vi "Create_Destination_for_Duplicate.vi"(8 "error in (no error)":errorcluster, 9 "subDirectory":string="data", 10 "Destinations in":refnum<class "AB_Destination.lvclass">[](array[class]), 11 "AB_Source_Library in":refnum<class "AB_Source_Library.lvclass">) -> (0 "error out":errorcluster, 1 "newPath":path, 2 "Destinations out":refnum<class "AB_Destination.lvclass">[](array[class]), 3 "AB_Source_Library out":refnum<class "AB_Source_Library.lvclass">)   [LabVIEW 2020, in "AB_Source_Library.lvclass"]
uses:
  <vilib>/AppBuilder/AB_Classes/Source/Library/AB_Source_Library.lvclass
  <vilib>/AppBuilder/AB_Classes/Destination/AB_Destination.lvclass
  e:/builds/penguin/labview/branches/2020/dev/dist/vi.lib/AppBuilder/AB_Classes/Source/AB_Source.lvclass
  <vilib>/AppBuilder/AB_Classes/Source/AB_Source.lvclass
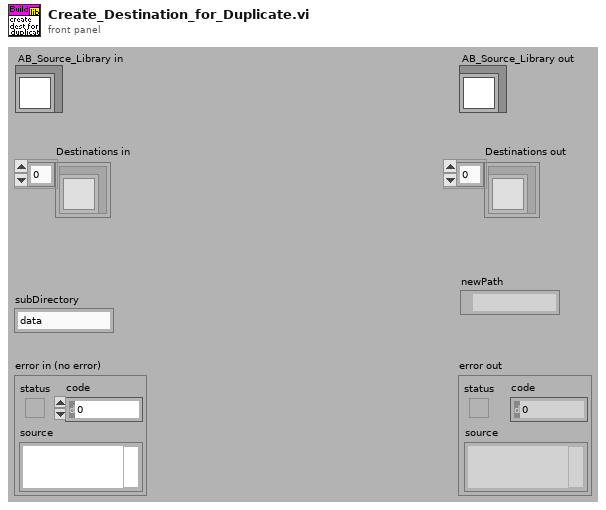
[diagram p1: front panel]
types:
  T1 = typedef "AB_Source.ctl" = cluster{"path":path, "itemID":string, "parentIndex":i32, "sourceInclusion":T2, "destinationIndex":i32, "properties":T3[], "newName":string, "lvfile":bool, "valid":bool, "eng_inBuild":bool, "eng_isNonVILink":bool, "Amalgamation":bool, "Amalgamation Piece":bool, "eng_delimitedName":string, "preventRename":bool}
  T2 = typedef "AB_Source_Inclusion.ctl" = enum16{"IncludeIfReferenced", "Include", "Exclude", "TopLevel"}
  T3 = typedef "AB_Source_Properties.ctl" = cluster{"sourcePropertyType":T4, "value":variant}
  T4 = typedef "AB_Source_Property_Type.ctl" = enum16{"Remove block diagram", "Remove front panel", "Password", "Window has title bar", "Show menu bar", "Show vertical scroll bar", "Show horizontal scroll bar", "Show toolbar", "Show Abort button", "Show fp when called", "Window behavior", "Allow user to close window", "Window run-time position", "Run when opened", "Allow debugging", "Auto error handling", "Generate guard code", "Use stack variables", "Expression folding", "Integer only", "Inline subVI"}
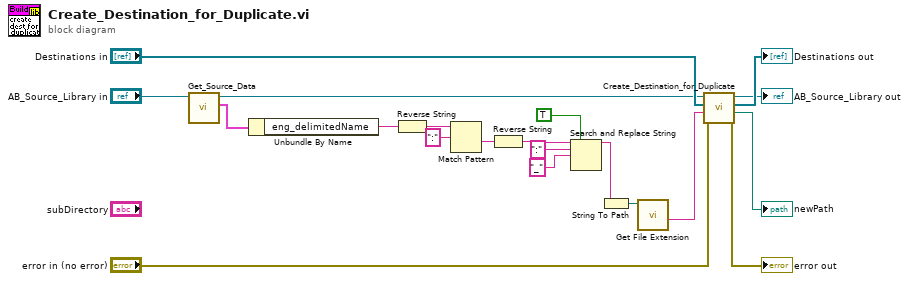
[diagram p0: block diagram]
diagram:
  n1 = call <vilib>:"Get_Source_Data.vi"("Class in"="AB_Source_Library in") -> ("data"=w1:T1, "Class out"=w2:refnum<class "AB_Source_Library.lvclass">)  [unwired: 8 in, 1 out]
  n2 = Unbundle By Name(w1) -> ("eng_delimitedName"=w10:string)
  n3 = Reverse String(1:w10) -> (0:w13:string)
  n4 = Match Pattern(string=w13, regular expression=":" ("search string/char (-)")) -> (after substring=w12:string)  [unwired: 1 in, 3 out]
  n5 = Reverse String(1:w12) -> (0:w9:string)
  n6 = Search and Replace String(replace all?=TRUE ("replace all? (F)"), input string=w9, search string=":", replace string="_" ("replace string (\"\")")) -> (result string=w8:string)  [unwired: 4 in, 3 out]
  n7 = String To Path(string=w8) -> (path=w11:path)
  n8 = call <vilib>:"Get File Extension.vi"("file"=w11) -> ("filename without extension"=w4:string)  [unwired: 6 in, 4 out]
  n9 = call-parent "Create_Destination_for_Duplicate.vi"("error in (no error)"="error in (no error)", "subDirectory"=w4, "Destinations in"="Destinations in", "AB_Source in"=w2) -> ("error out"=→"error out":errorcluster, "newPath"=→"newPath":path, "Destinations out"=→"Destinations out":refnum<class "AB_Destination.lvclass">[], "AB_Source out"=→"AB_Source_Library out":refnum<class "AB_Source_Library.lvclass">)  [unwired: 4 in]
